vi "Temperature Converter.vi"(7 "Direction":enum16{"F to C", "C to F"}(ring), 11 "In":dbl) -> (3 "Out":dbl)   [LabVIEW 2020]
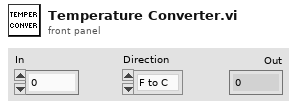
[diagram p1: front panel]
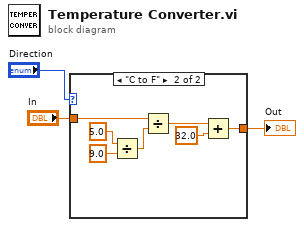
[diagram p0: block diagram]
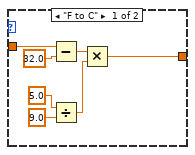
[diagram p2: hidden frame]
diagram:
  n1 = case shown="\"C to F\"" "Direction" {
    tunnel: "In" -> [w5 w13]
    tunnel: [w4 w14] -> w2
    frame "F to C" {
      n2 = Subtract(x=w5, y=32.0) -> (x-y=w6:dbl)
      n3 = Divide(x=5.0, y=9.0) -> (x/y=w7:dbl)
      n4 = Multiply(x=w6, y=w7) -> (x*y=w4:dbl)
    }
    frame "C to F" {
      n5 = Divide(x=5.0, y=9.0) -> (x/y=w12:dbl)
      n6 = Divide(x=w13, y=w12) -> (x/y=w11:dbl)
      n7 = Add(x=w11, y=32.0) -> (x+y=w14:dbl)
    }
  }
  "Out" <- w2
